vi "LC2_Global.vi"() -> ()   [LabVIEW 2016]
panel:
  out "LC2_WatchDogTimer_enable":bool
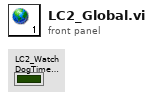
[diagram p1: front panel]
diagram:
